vi "Check if HSE Scripting Tools are installed.vi"(8 "error in":errorcluster) -> (0 "error out":errorcluster, 1 "HSE Scripting tools Installed?":bool)   [LabVIEW 2020, in "Panther Dashboard.lvlib"]
uses:
  Panther Dashboard.lvlib
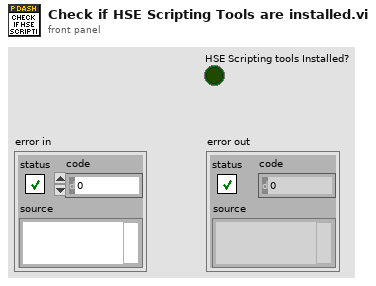
[diagram p1: front panel]
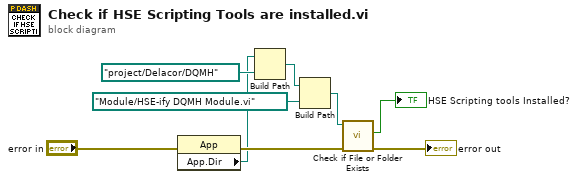
[diagram p0: block diagram]
diagram:
  n1 = property class="App"(error in="error in") -> (error out=w8:errorcluster, "App.Dir"=w4:path)  [unwired: 1 in, 1 out]
  n2 = Build Path(base path=w4, name or relative path=path "project/Delacor/DQMH" ("Application:Directory Path")) -> (appended path=w5:path)
  n3 = Build Path(base path=w5, name or relative path=path "Module/HSE-ify DQMH Module.vi") -> (appended path=w1:path)
  n4 = call <vilib>:"Check if File or Folder Exists.vi"("error in (no error)"=w8, "path"=w1) -> ("error out"=→"error out":errorcluster, "file or folder exists?"=→"HSE Scripting tools Installed?":bool)  [unwired: 7 in, 1 out]
